vi "testXbox.vi"() -> ()   [LabVIEW 2018]
uses:
  XInput9_1_0.dll
panel:
  out "Y":dbl
  out "X":dbl
  out "pState":T1
  out "XInput return":u32
  out "Buttons":T2
  out "연결됨?":bool
  in  "정지":bool
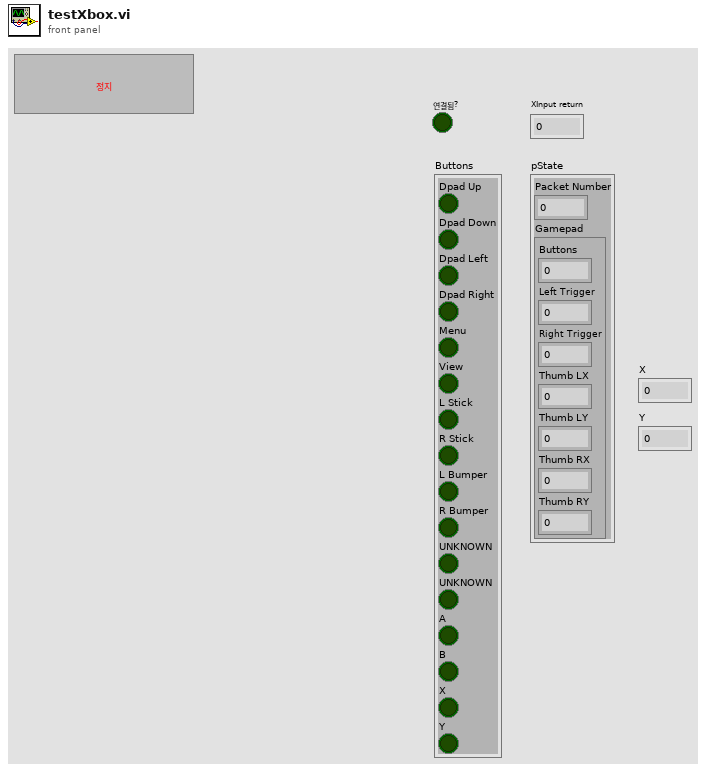
[diagram p1: front panel]
types:
  T1 = cluster{"Packet Number":u32, "Gamepad":cluster{"Buttons":u16, "Left Trigger":u8, "Right Trigger":u8, "Thumb LX":i16, "Thumb LY":i16, "Thumb RX":i16, "Thumb RY":i16}}
  T2 = cluster{"Dpad Up":bool, "Dpad Down":bool, "Dpad Left":bool, "Dpad Right":bool, "Menu":bool, "View":bool, "L Stick":bool, "R Stick":bool, "L Bumper":bool, "R Bumper":bool, "UNKNOWN":bool, "UNKNOWN":bool, "A":bool, "B":bool, "X":bool, "Y":bool}
  T3 = cluster{"Boolean array[0]":bool, "Boolean array[1]":bool, "Boolean array[2]":bool, "Boolean array[3]":bool, "Boolean array[4]":bool, "Boolean array[5]":bool, "Boolean array[6]":bool, "Boolean array[7]":bool, "Boolean array[8]":bool, "Boolean array[9]":bool, "Boolean array[10]":bool, "Boolean array[11]":bool, "Boolean array[12]":bool, "Boolean array[13]":bool, "Boolean array[14]":bool, "Boolean array[15]":bool}
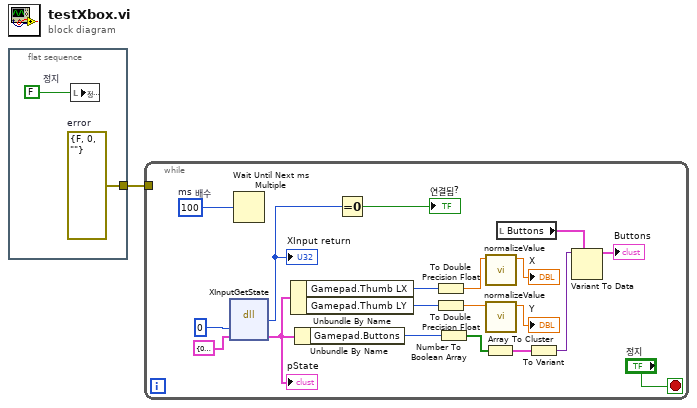
[diagram p0: block diagram]
diagram:
  n1 = flat-sequence {
    tunnel: [w3] -> w1
    frame #0 {
      w2 = FALSE  # 정지
      w3 = errorcluster {"status"=FALSE, "code"=0, "source"=""}  # error
      n2 = local write "정지"(w2) -> ()
    }
  }
  n3 = while {
    tunnel: w1 -> [_]
    stop <- "정지" stop-if-true
    w22 = u32 100  # ms 배수
    n4 = dll-call lib="XInput9_1_0.dll" fn="XInputGetState"("dwUserIndex"=u32 0, "pState"=T1 {"Packet Number"=0, "Gamepad"={"Buttons"=0, "Left Trigger"=0, "Right Trigger"=0, "Thumb LX"=0, "Thumb LY"=0, "Thumb RX"=0, "Thumb RY"=0}} ("XInput State")) -> ("return type"=w14:u32, "pState"=w10:T1)  [unwired: 4 in, 2 out]
    "XInput return" <- w14
    "pState" <- w10
    n5 = Wait Until Next ms Multiple(millisecond multiple=w22) -> ()  [unwired: 1 out]
    n6 = Unbundle By Name(w10) -> ("Gamepad.Thumb LX"=w9:i16, "Gamepad.Thumb LY"=w6:i16)
    n7 = Unbundle By Name(w10) -> ("Gamepad.Buttons"=w17:u16)
    n8 = Equal To 0?(x=w14) -> (x = 0?=→"연결됨?":bool)
    n9 = To Double Precision Float(number=w9) -> (double precision float=w8:dbl)
    n10 = To Double Precision Float(number=w6) -> (double precision float=w5:dbl)
    n11 = Number To Boolean Array(number=w17) -> (Boolean array=w15:bool[])
    n12 = Array To Cluster(array=w15) -> (cluster=w21:T3)
    n13 = call "normalizeValue.vi"("입력"=w8) -> ("출력"=→"X":dbl)  [unwired: 9 in, 1 out]
    n14 = call "normalizeValue.vi"("입력"=w5) -> ("출력"=→"Y":dbl)  [unwired: 9 in, 1 out]
    n15 = local read "Buttons"() -> (w16:T2)
    n16 = To Variant(anything=w21) -> (Variant=w20:variant)
    n17 = Variant To Data(type=w16, Variant=w20) -> (data=→"Buttons":T2)  [unwired: 1 in, 1 out]
  }
